vi "Server_to_python.vi"() -> ()   [LabVIEW 2021]
panel:
  out "error out":errorcluster
  out "Command\nreceived":string
  out "Iteration":i32
  out "String":string
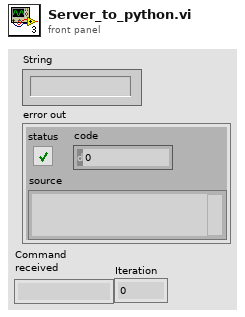
[diagram p1: front panel]
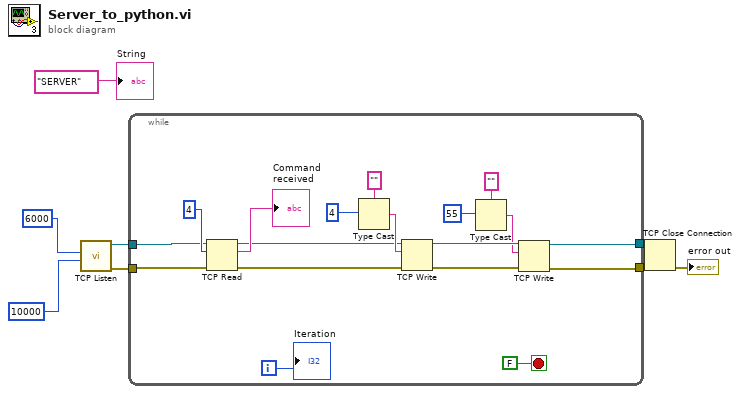
[diagram p0: block diagram]
diagram:
  n1 = call <vilib>:"TCP Listen.vi"("timeout ms (wait forever: -1)"=10000, "port"=u16 6000) -> ("error out"=w2:errorcluster, "connection ID"=w1:refnum<k5>)  [unwired: 5 in, 3 out]
  n2 = while {
    tunnel: [w12] -> w7
    tunnel: [w10] -> w6
    tunnel: w2 -> [w26]
    tunnel: w1 -> [w24]
    i -> [w23]
    stop <- FALSE stop-if-true
    n3 = TCP Read(connection ID=w24, bytes to read=4, error in (no error)=w26) -> (connection ID out=w18:refnum<k5>, data out=→"Command\nreceived":string, error out=w17:errorcluster)  [unwired: 2 in]
    n4 = Type Cast(type="", x=4) -> (*(type *) &x=w21:string)
    n5 = TCP Write(connection ID=w18, data in=w21, error in (no error)=w17) -> (connection ID out=w13:refnum<k5>, error out=w11:errorcluster)  [unwired: 1 in, 1 out]
    n6 = Type Cast(type="", x=55) -> (*(type *) &x=w9:string)
    n7 = TCP Write(connection ID=w13, data in=w9, error in (no error)=w11) -> (connection ID out=w12:refnum<k5>, error out=w10:errorcluster)  [unwired: 1 in, 1 out]
    "Iteration" <- w23
  }
  n8 = TCP Close Connection(connection ID=w7, error in (no error)=w6) -> (error out=→"error out":errorcluster)  [unwired: 1 in, 1 out]
  "String" <- "SERVER" ("String")
